vi "check_part_number_ref.vi"(4 "reload_part_number":string caption="Part Number:", 6 "reload_active?":bool, 8 "error_in":errorcluster, 11 "variable":variant) -> (0 "error_out":errorcluster, 2 "reload_part_number":string, 3 "gear_serial":string, 5 "part_number_ref_status":string)   [LabVIEW 2019]
uses:
  FGV/DOCK_records_display/FGV_DOCK_records_display.ctl
  _misc/AULocalize/SubVIs/Get Localized Phrase Compact Interface 0D.vi
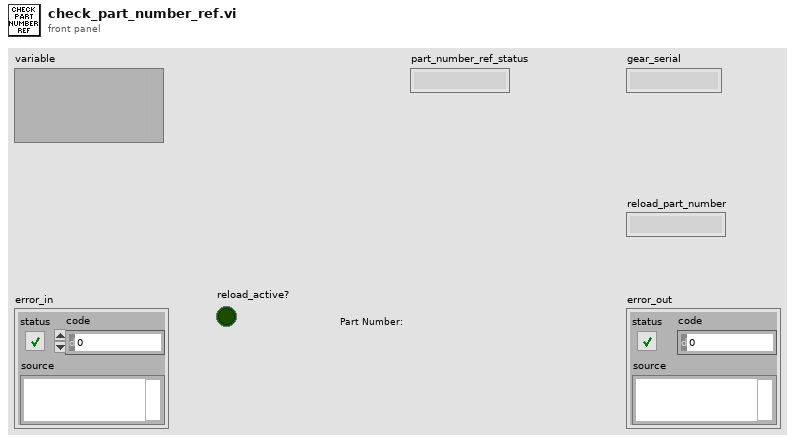
[diagram p1: front panel]
types:
  T1 = typedef "FGV_DOCK_records_display.ctl" = enum16{"initialize", "set_reference_data", "set_serial", "set_header", "set_operations", "set_results", "set_batches", "get_reference_data", "get_part_number_ref", "get_serial", "get_batch_code", "get_gear_ID", "get_operation_IDs", "toggle_results", "show_all_results", "hide_all_results", "display", "clear"}
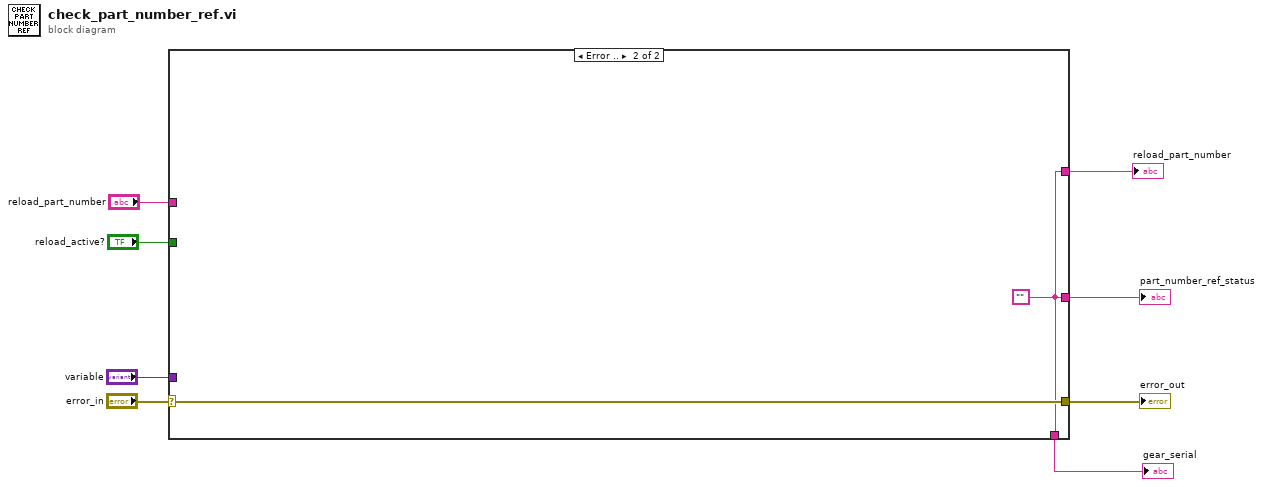
[diagram p0: block diagram]
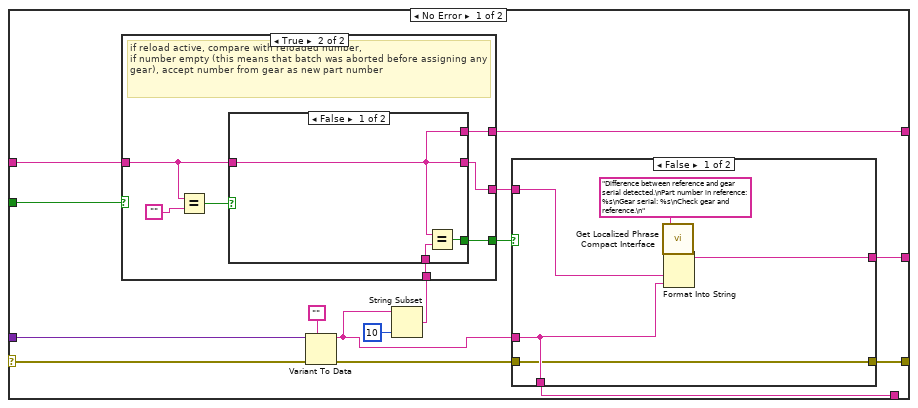
[diagram p2: hidden frame]
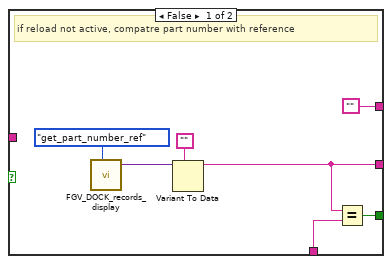
[diagram p3: hidden frame]
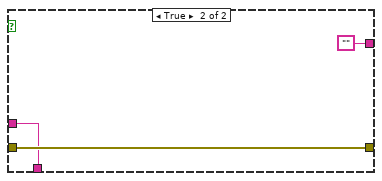
[diagram p5: hidden frame]
diagram:
  n1 = case shown="Error .." "error_in" {
    selector: "error_in" -> [w21 w54]
    tunnel: "variable" -> [w22 _]
    tunnel: [w18 w54] -> w6
    tunnel: [w17 w53] -> w5
    tunnel: [w14 w53] -> w4
    tunnel: "reload_active?" -> [w13 _]
    tunnel: "reload_part_number" -> [w12 _]
    tunnel: [w9 w53] -> w1
    frame No Error {
      n2 = Variant To Data(error in=w21, type="", Variant=w22) -> (data=w15:string, error out=w19:errorcluster)
      n3 = String Subset(string=w15, length (rest)=10 ("length (rest)")) -> (substring=w10:string)  [unwired: 1 in]
      n4 = case shown="True" w13 {
        tunnel: [w27 w35] -> w20
        tunnel: [w26 w31] -> w16
        tunnel: w12 -> [_ w32]
        tunnel: w10 -> [w25 w33]
        tunnel: ["" w34] -> w9
        frame False {
          # "if reload not active, compatre part number with reference"
          n5 = call "FGV_DOCK_records_display.vi"("options"=FGV_DOCK_records_display."get_part_number_ref") -> ("output"=w28:variant)  [unwired: 9 in, 1 out]
          n6 = Variant To Data(type="", Variant=w28) -> (data=w26:string)  [unwired: 1 in, 1 out]
          n7 = Equal?(x=w26, y=w25) -> (x = y?=w27:bool)
        }
        frame True {
          # "if reload active, compare with reloaded number,\nif number empty (this means that batch was aborted before assigning any gear), accept number from gear as new part number"
          n8 = Equal?(x=w32, y="") -> (x = y?=w36:bool)
          n9 = case shown="False" w36 {
            selector: w36 -> [_ w43]
            tunnel: [w39 w43] -> w35
            tunnel: [w38 w42] -> w34
            tunnel: w33 -> [w40 w42]
            tunnel: w32 -> [w38 w41]
            tunnel: [w38 w41] -> w31
            frame False {
              n10 = Equal?(x=w38, y=w40) -> (x = y?=w39:bool)
            }
            frame True {
            }
          }
        }
      }
      n11 = case shown="False" w20 {
        tunnel: w19 -> [w46 w52]
        tunnel: [w46 w52] -> w18
        tunnel: w15 -> [w47 w51]
        tunnel: [w47 w51] -> w17
        tunnel: w16 -> [w48 _]
        tunnel: [w45 ""] -> w14
        frame False {
          n12 = call-poly "Get Localized Phrase Compact Interface.vi"("Key"="Difference between reference and gear serial detected.\nPart number in reference: %s\nGear serial: %s\nCheck gear and reference.\n" ("format string")) -> ("Translated Phrase"=w44:string)
          n13 = Format Into String(format string=w44, w48, w47) -> (resulting string=w45:string)  [unwired: 2 in, 1 out]
        }
        frame True {
        }
      }
    }
    frame Error {
      w53 = ""
    }
  }
  "gear_serial" <- w5
  "error_out" <- w6
  "part_number_ref_status" <- w4
  "reload_part_number" <- w1
